vi "Create Reference Locals_Mod.vi"(5 "Sequence Context":refnum<k7>) -> (0 "error out":errorcluster)   [LabVIEW 2013, in "MiscHelperVIs.lvlib"]
uses:
  MiscHelperVIs.lvlib
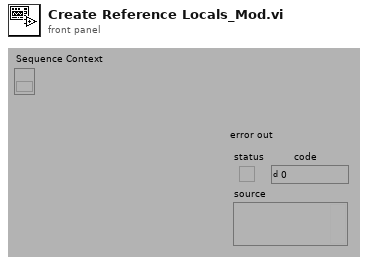
[diagram p1: front panel]
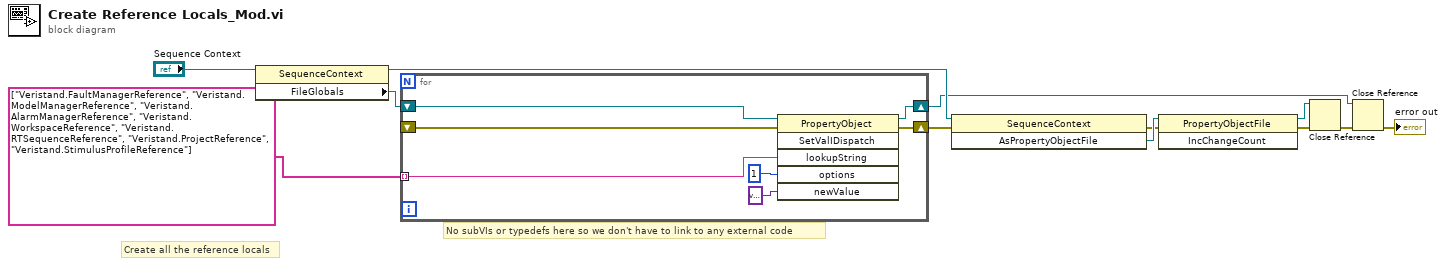
[diagram p0: block diagram]
diagram:
  # "No subVIs or typedefs here so we don't have to link to any external code"
  # "Create all the reference locals"
  n1 = property class="SequenceContext"(reference="Sequence Context") -> (reference out=w10:refnum<k7>, "FileGlobals"=w11:refnum<k7>)  [unwired: 1 in, 1 out]
  n2 = for {
    shift-right: [w15] -> w5
    shift-left: _ -> [w16]
    tunnel: string[] ["Veristand.FaultManagerReference", "Veristand.ModelManagerReference", "Veristand.AlarmManagerReference", "Veristand.WorkspaceReference", "Veristand.RTSequenceReference", "Veristand.ProjectReference", "Veristand.StimulusProfileReference"] -> [w18] mode=indexing
    shift-right: [w13] -> w4
    shift-left: w11 -> [w19]
    n3 = invoke class="PropertyObject" method="SetValIDispatch"(reference=w19, error in=w16, "lookupString"=w18, "options"=1, "newValue"=variant) -> (reference out=w13:refnum<k7>, error out=w15:errorcluster)  [unwired: 1 in, 4 out]
  }
  n4 = invoke class="SequenceContext" method="AsPropertyObjectFile"(reference=w10, error in=w5) -> (error out=w6:errorcluster, "AsPropertyObjectFile"=w9:refnum<k7>)  [unwired: 1 in, 1 out]
  n5 = invoke class="PropertyObjectFile" method="IncChangeCount"(reference=w9, error in=w6) -> (reference out=w8:refnum<k7>, error out=w7:errorcluster)  [unwired: 1 in, 1 out]
  n6 = Close Reference(reference=w8, error in (no error)=w7) -> (error out=w3:errorcluster)
  n7 = Close Reference(reference=w4, error in (no error)=w3) -> (error out=→"error out":errorcluster)
